vi "New - Add to Poly.vi"(6 "Selector Name":string, 7 "Poly Ref":refnum<vi>, 8 "error in (no error)":errorcluster, 9 "Menu Name":string, 10 "Path to VI":path, 11 "Poly Map Set in":T1) -> (0 "error out":errorcluster, 3 "Poly Map Set out":T1)   [LabVIEW 2020]
uses:
  _td_map_PolyInstanceInfo.ctl
  _td_cluster_InstanceInfo.ctl
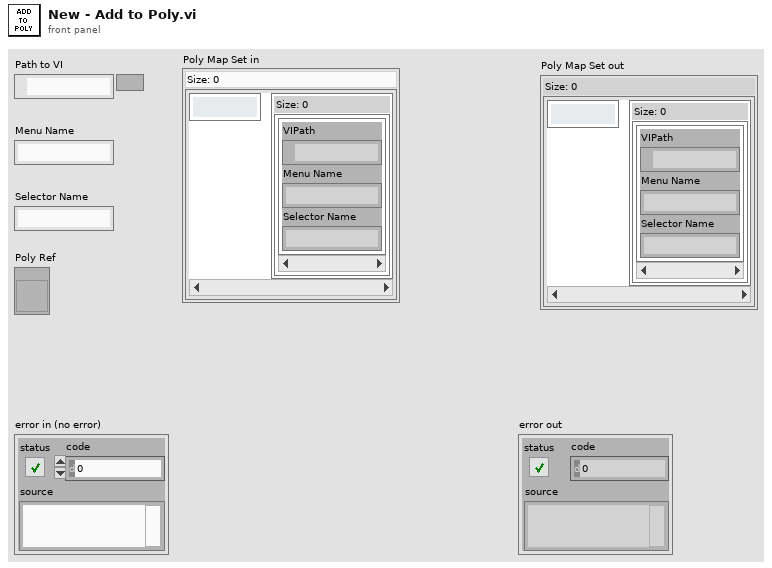
[diagram p1: front panel]
types:
  T1 = typedef "_td_map_PolyInstanceInfo.ctl" = map{string, set{T2}}
  T2 = typedef "_td_cluster_InstanceInfo.ctl" = cluster{"VIPath":path, "Menu Name":string, "Selector Name":string}
  T3 = cluster{"VIPath":path, "Menu Name":string, "Selector Name":string}
  T4 = cluster{"VIPath":path, "Menu Name":string, "Selector Name":string}[]
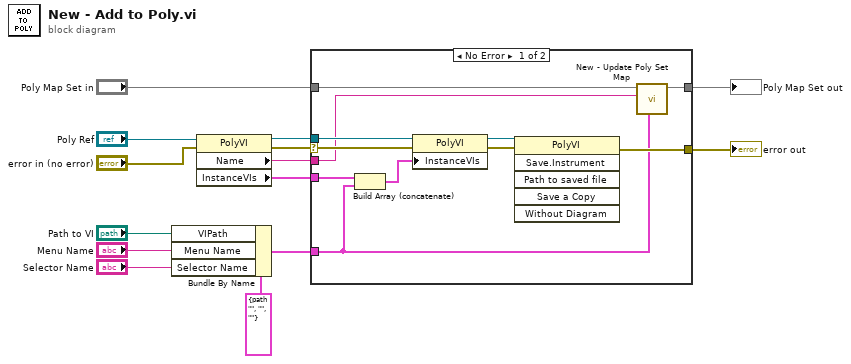
[diagram p0: block diagram]
diagram:
  n1 = Bundle By Name(cluster=T3 {"VIPath"=path "", "Menu Name"="", "Selector Name"=""}, "VIPath"="Path to VI", "Menu Name"="Menu Name", "Selector Name"="Selector Name") -> (w4:T3)
  n2 = property class="PolyVI"(reference="Poly Ref", error in="error in (no error)") -> (reference out=w11:refnum<vi>, error out=w12:errorcluster, "Name"=w10:string, "InstanceVIs"=w9:T4)
  n3 = case shown="No Error" w12 {
    selector: w12 -> [w23 w26]
    tunnel: w11 -> [w25 _]
    tunnel: w10 -> [w18 _]
    tunnel: w9 -> [w21 _]
    tunnel: w4 -> [w15 _]
    tunnel: "Poly Map Set in" -> [w19 w27]
    tunnel: [w17 w27] -> w2
    tunnel: [w16 w26] -> w1
    frame No Error {
      n4 = Build Array (concatenate)(w21, w15) -> (w20:T4)
      n5 = property class="PolyVI"(reference=w25, error in=w23, "InstanceVIs"=w20) -> (reference out=w24:refnum<vi>, error out=w22:errorcluster)
      n6 = invoke class="PolyVI" method="Save.Instrument"(reference=w24, error in=w22) -> (error out=w16:errorcluster)  [unwired: 4 in, 5 out]
      n7 = call "New - Update Poly Set Map.vi"("Instance Info"=w15, "Poly VI Name in"=w18, "Poly Map Set in"=w19) -> ("Poly Map Set out"=w17:T1)  [unwired: 7 in, 1 out]
    }
    frame Error {
    }
  }
  "Poly Map Set out" <- w2
  "error out" <- w1
